vi "UI_WindowFrame2.vi"() -> ()   [LabVIEW 2020]
uses:
  xcontrol/CloseXctl/CloseXctl.xctl
panel:
  out "Minimize":u16(ring)
  out "Maximize":u16(ring)
  out "Close":u16(ring)
  out "WindowTitle":bool
  in  "CloseXctl":bool(xcontrol)
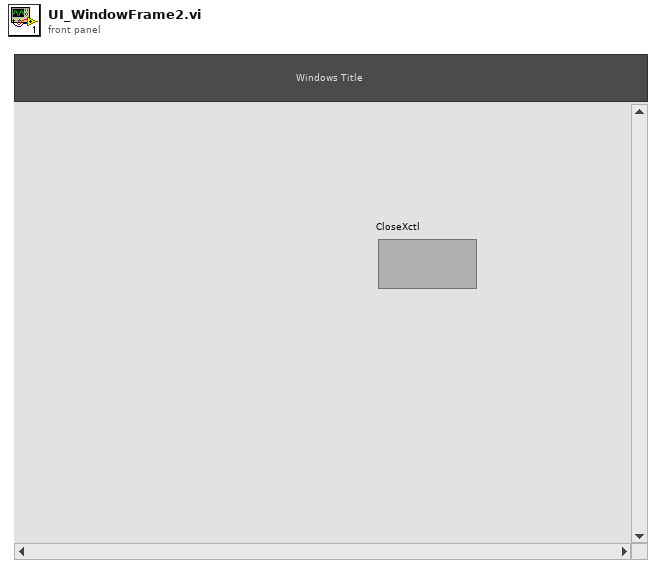
[diagram p1: front panel]
types:
  T1 = enum32{"Invalid", "Standard", "Closed", "Hidden", "Minimized", "Maximized"}
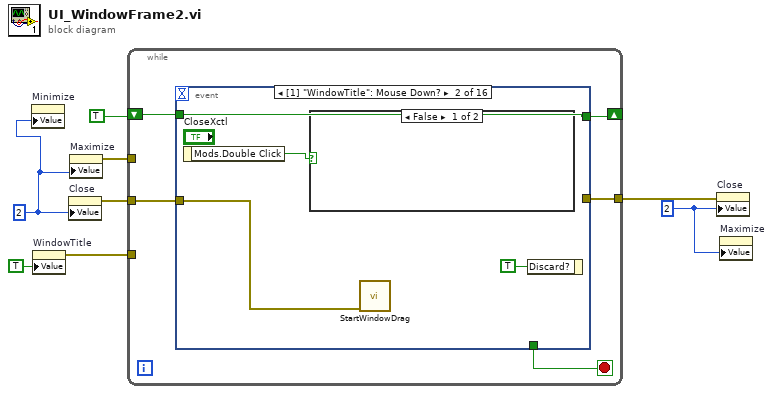
[diagram p0: block diagram]
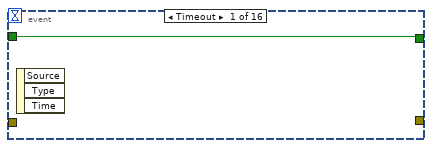
[diagram p2: hidden frame]
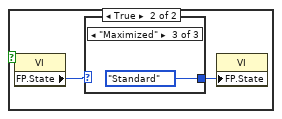
[diagram p3: hidden frame]
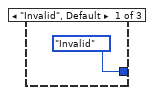
[diagram p4: hidden frame]
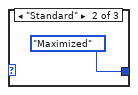
[diagram p5: hidden frame]
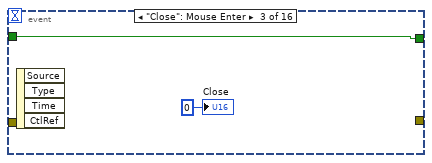
[diagram p6: hidden frame]
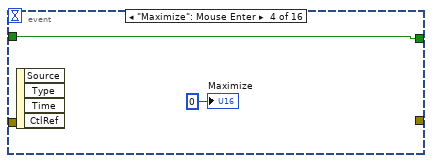
[diagram p7: hidden frame]
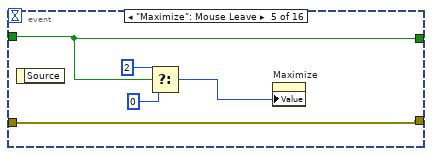
[diagram p8: hidden frame]
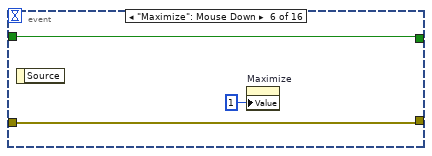
[diagram p9: hidden frame]
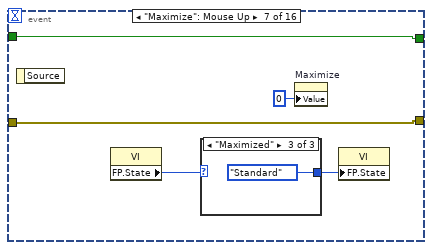
[diagram p10: hidden frame]
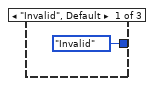
[diagram p11: hidden frame]
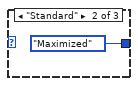
[diagram p12: hidden frame]
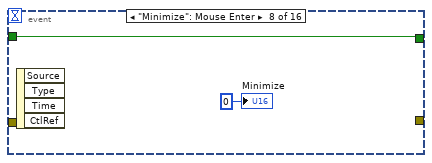
[diagram p13: hidden frame]
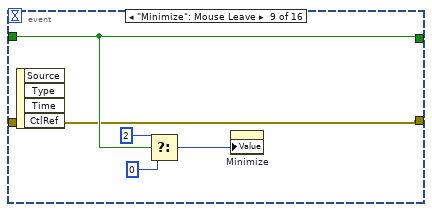
[diagram p14: hidden frame]
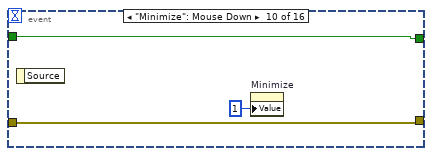
[diagram p15: hidden frame]
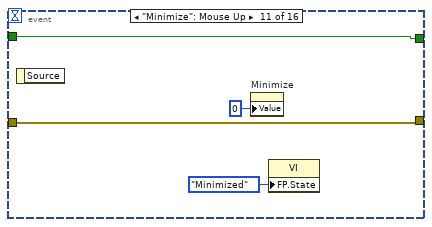
[diagram p16: hidden frame]
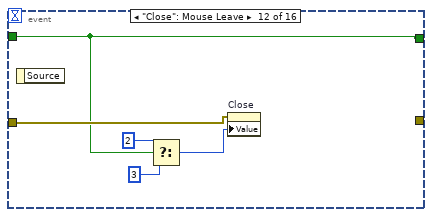
[diagram p17: hidden frame]
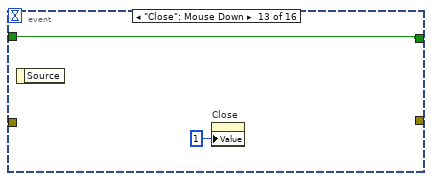
[diagram p18: hidden frame]
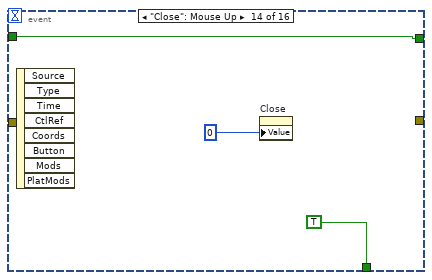
[diagram p19: hidden frame]
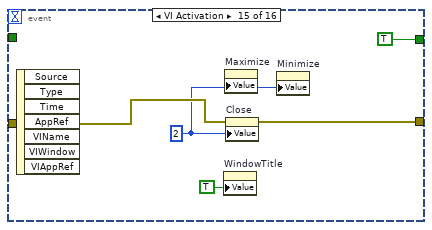
[diagram p20: hidden frame]
diagram:
  w2 = u16 2 ("Close")
  w1 = u16 2 ("Close")
  n1 = property on="Minimize" class="Ring (strict)"("Value"=w1) -> ()  [unwired: 2 in, 2 out]
  n2 = property on="WindowTitle" class="Bool (strict)"("Value"=TRUE ("WindowTitle")) -> (error out=w6:errorcluster)  [unwired: 2 in, 1 out]
  n3 = property on="Close" class="Ring (strict)"("Value"=w1) -> (error out=w8:errorcluster)  [unwired: 2 in, 1 out]
  n4 = property on="Maximize" class="Ring (strict)"("Value"=w1) -> (error out=w3:errorcluster)  [unwired: 2 in, 1 out]
  n5 = while {
    tunnel: w8 -> [w13]
    tunnel: w6 -> [_]
    shift-right: [w10] -> _
    shift-left: TRUE -> [w11]
    tunnel: [w9] -> w4
    tunnel: w3 -> [_]
    stop <- w12 stop-if-true
    n6 = event shown="[1] \"WindowTitle\": Mouse Down?" {
      selector: _ -> [_ _ _ _ _ _ _ _ _ _ _ _ _ _ _ _]
      dyn-events: _ -> [_ _ _ _ _ _ _ _ _ _ _ _ _ _ _ _]
      timeout: _ -> [_ _ _ _ _ _ _ _ _ _ _ _ _ _ _ _]
      tunnel: w13 -> [_ w17 _ _ w32 w33 w40 _ w46 w51 w55 w62 _ _ w70 _]
      tunnel: [_ _ _ _ _ _ _ _ _ _ _ _ _ TRUE _ _] -> w12
      tunnel: w11 -> [w14 w16 w24 w26 w28 w35 w39 w44 w47 w53 w57 w58 w63 w65 _ _]
      tunnel: [w14 w16 w24 w26 w28 w35 w39 w44 w47 w53 w57 w58 w63 w65 TRUE FALSE] -> w10
      tunnel: [_ _ _ _ w32 w33 w40 _ w46 w51 w55 _ _ _ w69 _] -> w9
      event Timeout {
        n7 = event-data() -> ()  [unwired: 1 in, 3 out]
      }
      event "WindowTitle": Mouse Down? {
        n8 = event-data() -> ("Mods.Double Click"=w15:bool)  [unwired: 1 in]
        n9 = case shown="False" w15 {
          frame False {
          }
          frame True {
            n10 = property class="VI"() -> ("FP.State"=w19:T1)  [unwired: 2 in, 2 out]
            n11 = case shown="\"Maximized\"" w19 {
              tunnel: [T1."Invalid" ("Front Panel Window:State") T1."Maximized" ("Front Panel Window:State") T1."Standard" ("Front Panel Window:State")] -> w20
              frame "Invalid", Default {
              }
              frame "Standard" {
              }
              frame "Maximized" {
              }
            }
            n12 = property class="VI"("FP.State"=w20) -> ()  [unwired: 2 in, 2 out]
          }
        }
        n13 = call "StartWindowDrag.vi"("error in (no error)"=w17) -> ()  [unwired: 9 in, 2 out]
        n14 = event-data("Discard?"=TRUE) -> ()  [unwired: 1 in, 1 out]
      }
      event "Close": Mouse Enter {
        n15 = event-data() -> ()  [unwired: 1 in, 4 out]
        "Close" <- u16 0 ("Close")
      }
      event "Maximize": Mouse Enter {
        n16 = event-data() -> ()  [unwired: 1 in, 4 out]
        "Maximize" <- u16 0 ("Maximize")
      }
      event "Maximize": Mouse Leave {
        n17 = event-data() -> ()  [unwired: 1 in, 1 out]
        n18 = Select(t=u16 2 ("Close"), s=w28, f=u16 0 ("Close")) -> (s? t:f=w29:u16)
        n19 = property on="Maximize" class="Ring (strict)"("Value"=w29) -> ()  [unwired: 2 in, 2 out]
      }
      event "Maximize": Mouse Down {
        n20 = event-data() -> ()  [unwired: 1 in, 1 out]
        n21 = property on="Maximize" class="Ring (strict)"("Value"=u16 1 ("Maximize")) -> ()  [unwired: 2 in, 2 out]
      }
      event "Maximize": Mouse Up {
        n22 = event-data() -> ()  [unwired: 1 in, 1 out]
        n23 = property class="VI"() -> ("FP.State"=w36:T1)  [unwired: 2 in, 2 out]
        n24 = case shown="\"Maximized\"" w36 {
          tunnel: [T1."Invalid" ("Front Panel Window:State") T1."Maximized" ("Front Panel Window:State") T1."Standard" ("Front Panel Window:State")] -> w37
          frame "Invalid", Default {
          }
          frame "Standard" {
          }
          frame "Maximized" {
          }
        }
        n25 = property on="Maximize" class="Ring (strict)"("Value"=u16 0 ("Maximize")) -> ()  [unwired: 2 in, 2 out]
        n26 = property class="VI"("FP.State"=w37) -> ()  [unwired: 2 in, 2 out]
      }
      event "Minimize": Mouse Enter {
        n27 = event-data() -> ()  [unwired: 1 in, 4 out]
        "Minimize" <- u16 0 ("Minimize")
      }
      event "Minimize": Mouse Leave {
        n28 = event-data() -> ()  [unwired: 1 in, 4 out]
        n29 = Select(t=u16 2 ("Close"), s=w47, f=u16 0 ("Close")) -> (s? t:f=w48:u16)
        n30 = property on="Minimize" class="Ring (strict)"("Value"=w48) -> ()  [unwired: 2 in, 2 out]
      }
      event "Minimize": Mouse Down {
        n31 = event-data() -> ()  [unwired: 1 in, 1 out]
        n32 = property on="Minimize" class="Ring (strict)"("Value"=u16 1 ("Minimize")) -> ()  [unwired: 2 in, 2 out]
      }
      event "Minimize": Mouse Up {
        n33 = event-data() -> ()  [unwired: 1 in, 1 out]
        n34 = property on="Minimize" class="Ring (strict)"("Value"=u16 0 ("Minimize")) -> ()  [unwired: 2 in, 2 out]
        n35 = property class="VI"("FP.State"=T1."Minimized" ("Front Panel Window:State")) -> ()  [unwired: 2 in, 2 out]
      }
      event "Close": Mouse Leave {
        n36 = event-data() -> ()  [unwired: 1 in, 1 out]
        n37 = Select(t=u16 2 ("Close"), s=w58, f=u16 3 ("Close")) -> (s? t:f=w61:u16)
        n38 = property on="Close" class="Ring (strict)"(error in=w62, "Value"=w61) -> ()  [unwired: 1 in, 2 out]
      }
      event "Close": Mouse Down {
        n39 = event-data() -> ()  [unwired: 1 in, 1 out]
        n40 = property on="Close" class="Ring (strict)"("Value"=u16 1 ("Close")) -> ()  [unwired: 2 in, 2 out]
      }
      event "Close": Mouse Up {
        n41 = event-data() -> ()  [unwired: 1 in, 8 out]
        n42 = property on="Close" class="Ring (strict)"("Value"=u16 0 ("Close")) -> ()  [unwired: 2 in, 2 out]
      }
      event VI Activation {
        w68 = u16 2 ("Close")
        n43 = event-data() -> ()  [unwired: 1 in, 7 out]
        n44 = property on="WindowTitle" class="Bool (strict)"("Value"=TRUE ("WindowTitle")) -> ()  [unwired: 2 in, 2 out]
        n45 = property on="Maximize" class="Ring (strict)"("Value"=w68) -> ()  [unwired: 2 in, 2 out]
        n46 = property on="Close" class="Ring (strict)"(error in=w70, "Value"=w68) -> (error out=w69:errorcluster)  [unwired: 1 in, 1 out]
        n47 = property on="Minimize" class="Ring (strict)"("Value"=w68) -> ()  [unwired: 2 in, 2 out]
      }
      event event #0x53 {
        w73 = u16 0 ("Maximize")
        n48 = event-data() -> ()  [unwired: 1 in, 1 out]
        n49 = property on="Close" class="Ring (strict)"("Value"=u16 3 ("Close")) -> ()  [unwired: 2 in, 2 out]
        n50 = property on="Maximize" class="Ring (strict)"("Value"=w73) -> ()  [unwired: 2 in, 2 out]
        n51 = property on="Minimize" class="Ring (strict)"("Value"=w73) -> ()  [unwired: 2 in, 2 out]
        "WindowTitle" <- FALSE ("WindowTitle")
      }
    }
  }
  n52 = property on="Close" class="Ring (strict)"(error in=w4, "Value"=w2) -> ()  [unwired: 1 in, 2 out]
  n53 = property on="Maximize" class="Ring (strict)"("Value"=w2) -> ()  [unwired: 2 in, 2 out]
